vi "Panic on Error.vi"(3 "error in (no error)":errorcluster) -> ()   [LabVIEW 2018, in "Utilities.lvlib"]
uses:
  Utilities.lvlib
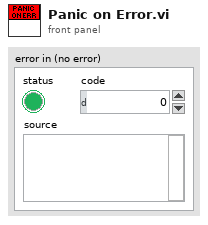
[diagram p1: front panel]
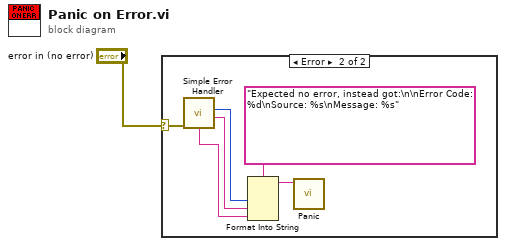
[diagram p0: block diagram]
diagram:
  n1 = case shown="Error" "error in (no error)" {
    selector: "error in (no error)" -> [_ w7]
    frame No Error {
    }
    frame Error {
      n2 = call <vilib>:"Simple Error Handler.vi"("error in (no error)"=w7) -> ("code out"=w5:i32, "source out"=w4:string, "message"=w3:string)  [unwired: 4 in, 2 out]
      n3 = Format Into String(format string="Expected no error, instead got:\n\nError Code: %d\nSource: %s\nMessage: %s", w5, w4, w3) -> (resulting string=w2:string)  [unwired: 2 in, 1 out]
      n4 = call "Panic.vi"("message (\"\")"=w2) -> ()  [unwired: 11 in]
    }
  }
